vi "Find All Children.vi"(8 "error in (no error)":errorcluster, 9 "Panel":string) -> (0 "error out":errorcluster, 2 "All Children":string[](array[string]))   [LabVIEW 2019, in "Panel.lvlib" / "Panel Registry.lvclass"]
uses:
  <vilib>/MGI/Panel Manager/Panel/Panel Registry/Panel Registry.lvclass
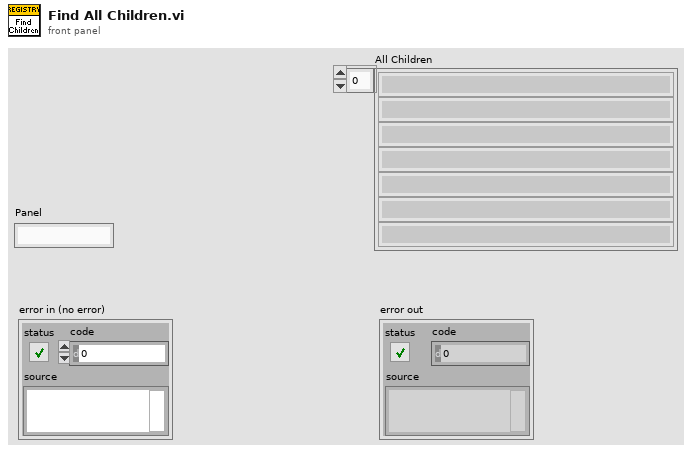
[diagram p1: front panel]
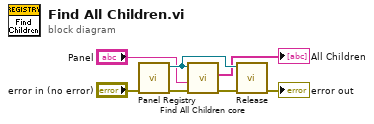
[diagram p0: block diagram]
diagram:
  n1 = call <vilib>:"Panel Registry.vi"("error in (no error)"="error in (no error)") -> ("error out"=w7:errorcluster, "Panel Registry out"=w5:refnum<class "Panel Registry.lvclass">)  [unwired: 9 in]
  n2 = call <vilib>:"Find All Children core.vi"("error in (no error)"=w7, "Panel"="Panel", "Panel Registry in"=w5) -> ("error out"=w6:errorcluster, "All Children"=→"All Children":string[])  [unwired: 7 in]
  n3 = call <vilib>:"Release.vi"("error in (no error)"=w6, "Panel Registry in"=w5) -> ("error out"=→"error out":errorcluster)  [unwired: 9 in]
